vi "HostSolenoidIndicators (1).vi"(11 "Array in":bool[](array[boolean])) -> (2 "Right Solenoids":cluster{string, bool}[](array[cluster]), 3 "Left Solenoids":cluster{string, bool}[](array[cluster]))   [LabVIEW 2017]
uses:
  RTControl/SolenoidsIndex.ctl
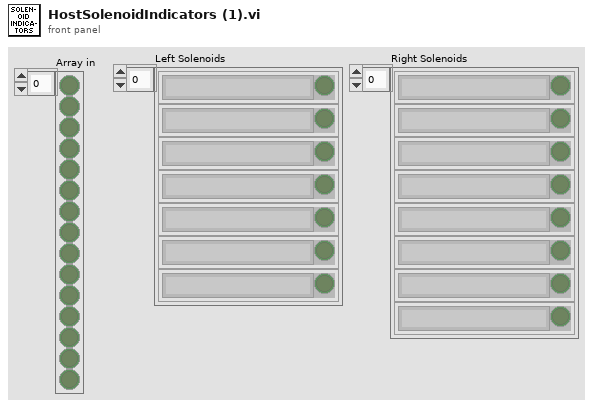
[diagram p1: front panel]
types:
  T1 = typedef "SolenoidsIndex.ctl" = enum16{"NC03", "NC04", "NC02", "NC10 MagIn", "NO02 MagOut", "NC01", "Pod Power", "NC09 SuspIn", "NO01 SuspOut", "NC08", "NC05", "NC06", "NC07", "NO03 AllOut", "Safety Panel Indicator"}
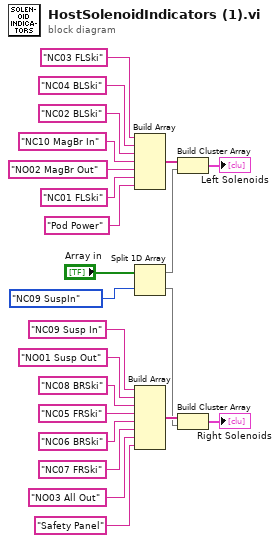
[diagram p0: block diagram]
diagram:
  n1 = Build Array("NC03 FLSki", "NC04 BLSki", "NC02 BLSki", "NC10 MagBr In", "NO02 MagBr Out", "NC01 FLSki", "Pod Power") -> (w16:string[])
  n2 = Split 1D Array(array="Array in", index=SolenoidsIndex."NC09 SuspIn" ("SolenoidsIndex")) -> (first subarray=w11:bool[], second subarray=w10:bool[])
  n3 = Build Array("NC09 Susp In", "NO01 Susp Out", "NC08 BRSki", "NC05 FRSki", "NC06 BRSki", "NC07 FRSki", "NO03 All Out", "Safety Panel") -> (w14:string[])
  n4 = Build Cluster Array(w16, w11) -> (→"Left Solenoids":cluster{string, bool}[])
  n5 = Build Cluster Array(w14, w10) -> (→"Right Solenoids":cluster{string, bool}[])
